vi "Endurance Pattern Paths.vi"(8 "error in (no error)":errorcluster, 11 "i":i32) -> (0 "error out":errorcluster, 2 "reset path":path, 3 "set path":path)   [LabVIEW 2018]
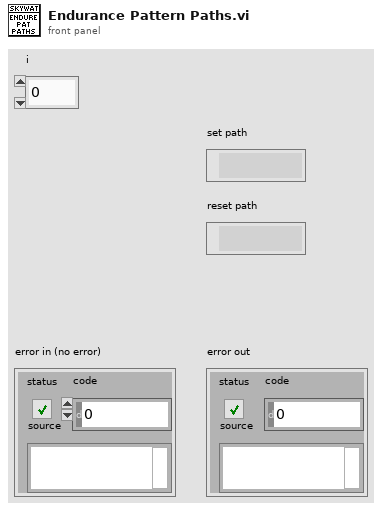
[diagram p1: front panel]
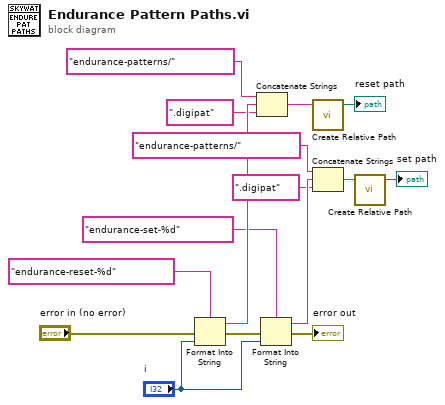
[diagram p0: block diagram]
diagram:
  n1 = Format Into String(format string="endurance-reset-%d" ("start label"), error in="error in (no error)", "i") -> (resulting string=w13:string, error out=w3:errorcluster)  [unwired: 1 in]
  n2 = Concatenate Strings("endurance-patterns/" ("string"), w13, ".digipat" ("string")) -> (w7:string)
  n3 = Format Into String(format string="endurance-set-%d" ("start label"), error in=w3, "i") -> (resulting string=w14:string, error out=→"error out":errorcluster)  [unwired: 1 in]
  n4 = call "Create Relative Path.vi"("file name"=w7) -> ("appended path"=→"reset path":path)  [unwired: 4 in]
  n5 = Concatenate Strings("endurance-patterns/" ("string"), w14, ".digipat" ("string")) -> (w11:string)
  n6 = call "Create Relative Path.vi"("file name"=w11) -> ("appended path"=→"set path":path)  [unwired: 4 in]
